vi "UsrProfiles-Profiles shortcut activ handler.vi"(8 "error in":errorcluster, 9 "Coords":T1, 10 "Users ListBox MenuRef":refnum<k9>, 11 "Users ListBox ref":refnum<vi>) -> (0 "error out":errorcluster)   [LabVIEW 2020]
uses:
  <vilib>/Utility/miscctls.llb/LVPoint32TypeDef.ctl
  Typedefs/Which path.ctl
  Globals/gl_UsrProfiles globals.vi
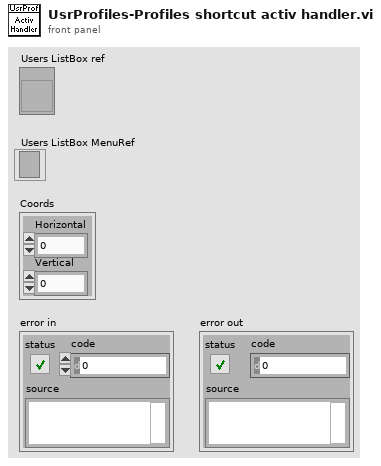
[diagram p1: front panel]
types:
  T1 = typedef "LVPoint32TypeDef.ctl" = cluster{"Horizontal":i32, "Vertical":i32}
  T2 = typedef "Which path.ctl" = enum16{"Configuration Files", "Calibration Files", "Images", "Setup.ini", "Loaded User profile.ini", "User's-Previous session.ini", "New user profile.ini", "Selected User profile.ini", "User profiles folder", "Power meter scaling.txt", "FOV Cal.ini", "Calibration.ini"}
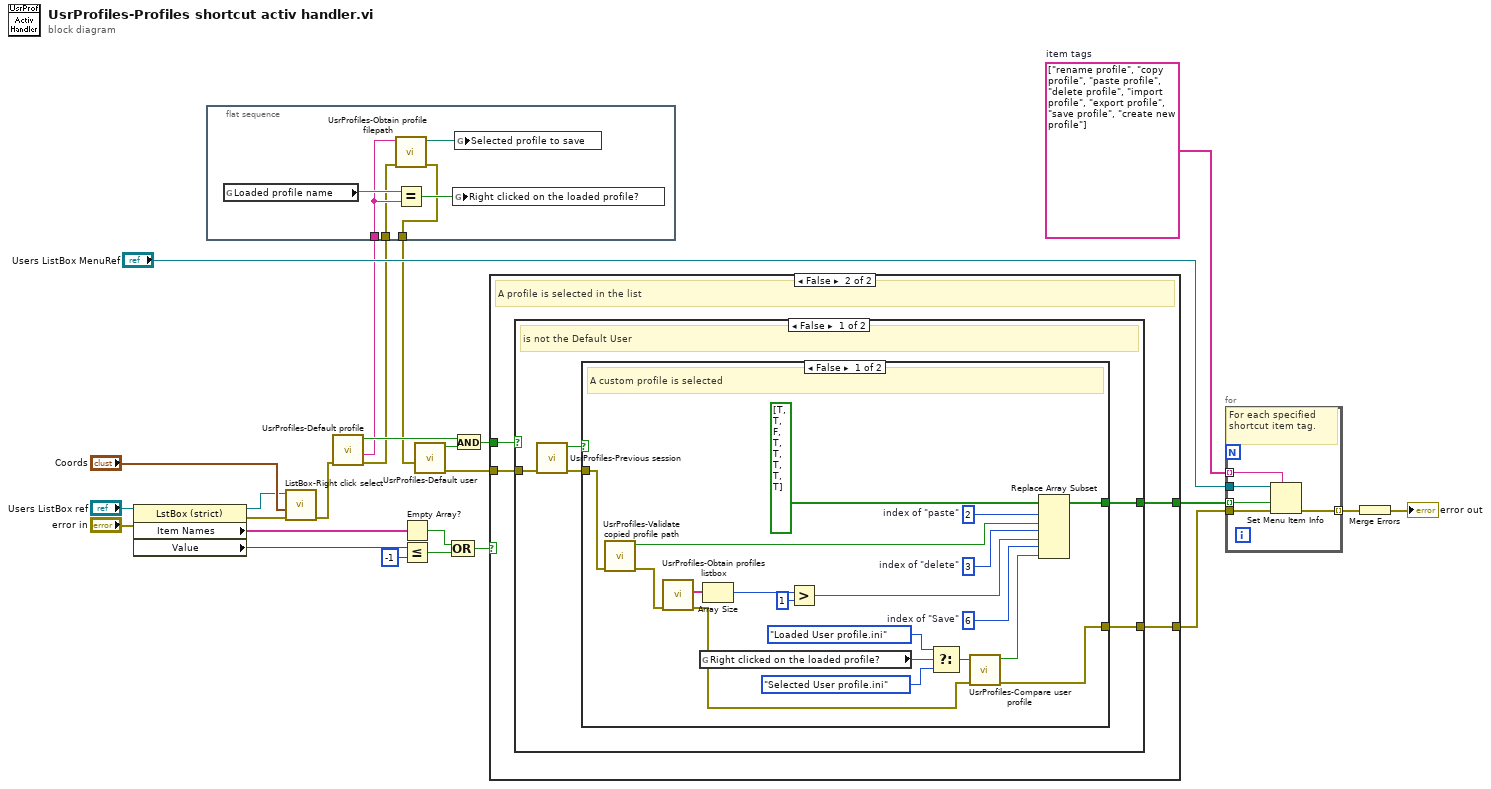
[diagram p0: block diagram]
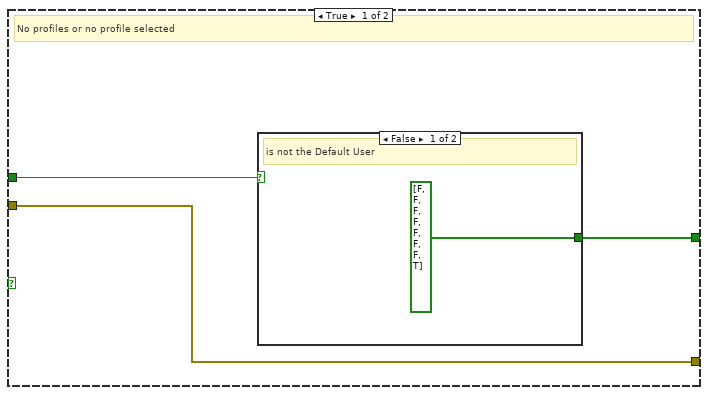
[diagram p2: hidden frame]
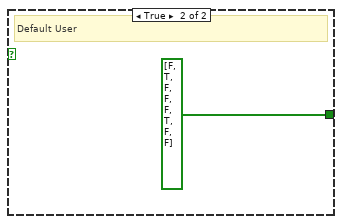
[diagram p3: hidden frame]
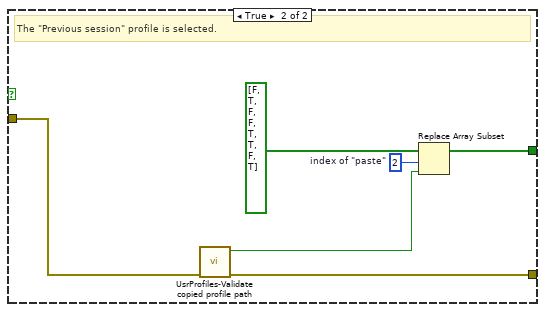
[diagram p4: hidden frame]
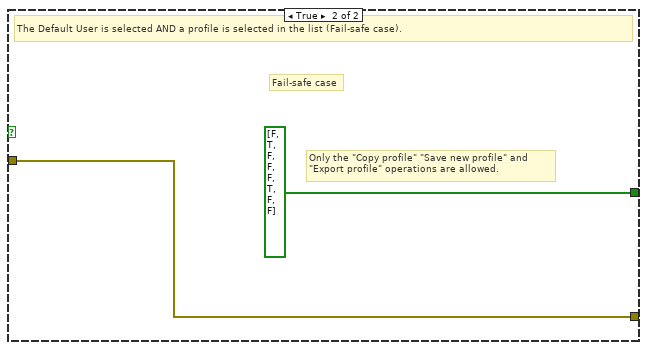
[diagram p5: hidden frame]
diagram:
  w20 = string[] ["rename profile", "copy profile", "paste profile", "delete profile", "import profile", "export profile", "save profile", "create new profile"]  # item tags
  n1 = property on="Property Node" class="LstBox (strict)"(reference="Users ListBox ref", error in="error in") -> (reference out=w8:refnum<vi>, error out=w7:errorcluster, "Item Names"=w9:string[], "Value"=w18:i32)
  n2 = flat-sequence {
    tunnel: w3 -> [w28]
    tunnel: [w26] -> w1
    tunnel: w2 -> [w27]
    frame #0 {
      n3 = global read "gl_UsrProfiles globals.vi" "Loaded profile name"() -> (w31:string)
      n4 = call "UsrProfiles-Obtain profile filepath.vi"("error in"=w27, "Profile name"=w28) -> ("error out"=w26:errorcluster, "Profile filepath"=w29:path)  [unwired: 8 in]
      n5 = Equal?(x=w31, y=w28) -> (x = y?=w30:bool)
      n6 = global write "gl_UsrProfiles globals.vi" "Right clicked on the loaded profile?"(w30) -> ()
      n7 = global write "gl_UsrProfiles globals.vi" "Selected profile to save"(w29) -> ()
    }
  }
  n8 = call <userlib>:"ListBox-Right click select.vi"("error in"=w7, "Coords"="Coords", "ListBox ref"=w8) -> ("error out"=w5:errorcluster)  [unwired: 7 in, 1 out]
  n9 = call "UsrProfiles-Default profile.vi"("error in (no error)"=w5) -> ("error out"=w2:errorcluster, "Selected profile's name"=w3:string, "Default profile selected"=w13:bool)  [unwired: 8 in]
  n10 = Empty Array?(array=w9) -> (empty?=w15:bool)
  n11 = Less Or Equal?(x=w18, y=-1) -> (x <= y?=w16:bool)
  n12 = call "UsrProfiles-Default user.vi"("error in (no error)"=w1) -> ("error out"=w4:errorcluster, "Default user selected"=w12:bool)  [unwired: 8 in, 1 out]
  n13 = Compound Arithmetic op=OR(w15, w16) -> (w14:bool)
  n14 = And(x=w13, y=w12) -> (x .and. y?=w11:bool)
  n15 = case shown="False" w14 {
    tunnel: [w33 w40] -> w19
    tunnel: w11 -> [w34 w39]
    tunnel: [w32 w38] -> w6
    tunnel: w4 -> [w32 w37]
    frame True {
      # "No profiles or no profile selected"
      n16 = case shown="False" w34 {
        tunnel: [bool[] [FALSE, FALSE, FALSE, FALSE, FALSE, FALSE, FALSE, TRUE] bool[] [FALSE, TRUE, FALSE, FALSE, FALSE, TRUE, FALSE, FALSE]] -> w33
        frame False {
          # "is not the Default User"
        }
        frame True {
          # "Default User"
        }
      }
    }
    frame False {
      # "A profile is selected in the list"
      n17 = case shown="False" w39 {
        tunnel: [w45 bool[] [FALSE, TRUE, FALSE, FALSE, FALSE, TRUE, FALSE, FALSE]] -> w40
        tunnel: [w44 w71] -> w38
        tunnel: w37 -> [w42 w71]
        frame False {
          # "is not the Default User"
          n18 = call "UsrProfiles-Previous session.vi"("error in (no error)"=w42) -> ("error out"=w41:errorcluster, "Previous session profile selected"=w43:bool)  [unwired: 9 in]
          n19 = case shown="False" w43 {
            tunnel: [w63 w69] -> w45
            tunnel: [w53 w65] -> w44
            tunnel: w41 -> [w54 w66]
            frame False {
              w51 = 6  # index of "Save"
              w57 = 3  # index of "delete"
              w62 = 2  # index of "paste"
              # "A custom profile is selected"
              n20 = call "UsrProfiles-Validate copied profile path.vi"("error in"=w54) -> ("error out"=w55:errorcluster, "copied profile file still exists"=w61:bool)  [unwired: 8 in, 1 out]
              n21 = call "UsrProfiles-Obtain profiles listbox.vi"("error in (no error)"=w55) -> ("error out"=w46:errorcluster, "Profiles"=w60:string[])  [unwired: 7 in, 2 out]
              n22 = global read "gl_UsrProfiles globals.vi" "Right clicked on the loaded profile?"() -> (w48:bool)
              n23 = Array Size(array=w60) -> (size(s)=w59:i32)
              n24 = Greater?(x=w59, y=1) -> (0:w56:bool)
              n25 = Select(t=Which_path."Loaded User profile.ini" ("Which file?"), s=w48, f=Which_path."Selected User profile.ini" ("Which file?")) -> (s? t:f=w47:T2)
              n26 = call "UsrProfiles-Compare user profile.vi"("error in"=w46, "Which profile?"=w47) -> ("error out"=w53:errorcluster, "Changes exist"=w52:bool)  [unwired: 8 in]
              n27 = Replace Array Subset(array=bool[] [TRUE, TRUE, FALSE, TRUE, TRUE, TRUE, TRUE, TRUE], new element #1=w61, index #1=w62, new element #2=w56, index #2=w57, new element #3=w52, index #3=w51) -> (w63:bool[])
            }
            frame True {
              w68 = 2  # index of "paste"
              # "The \"Previous session\" profile is selected."
              n28 = call "UsrProfiles-Validate copied profile path.vi"("error in"=w66) -> ("error out"=w65:errorcluster, "copied profile file still exists"=w67:bool)  [unwired: 8 in, 1 out]
              n29 = Replace Array Subset(array=bool[] [FALSE, TRUE, FALSE, FALSE, TRUE, TRUE, FALSE, TRUE], new element=w67, index=w68) -> (w69:bool[])
            }
          }
        }
        frame True {
          # "Fail-safe case"
          # "Only the \"Copy profile\" \"Save new profile\" and\n\"Export profile\" operations are allowed."
          # "The Default User is selected AND a profile is selected in the list (Fail-safe case)."
        }
      }
    }
  }
  n30 = for {
    tunnel: "Users ListBox MenuRef" -> [w77]
    tunnel: w6 -> [w76]
    tunnel: [w75] -> w21 mode=indexing
    tunnel: w20 -> [w74] mode=indexing
    tunnel: w19 -> [w73] mode=indexing
    # "For each specified shortcut item tag."
    n31 = Set Menu Item Info(7:w74, 8:w76, 9:w73, 11:w77) -> (0:w75:errorcluster)  [unwired: 3 in, 1 out]
  }
  n32 = Merge Errors(w21) -> (→"error out":errorcluster)
